vi "Get Waveform Queue Settings.vi"(1 "RT Data in":T1={"Device Ref"=18446744073709551615, "Waveforms"=[], "Channels"={"Command Chan Refs"=[], "Command Data Refs"=[], "Command Values"=[], "Status Chan Refs"=[], "Status Data Refs"=[], "Status Values"=[], "System Time"={"System Time"=timestamp(0 s since 1904-01-01), "Data Reference"=0, "Absolute Time Channel Data Ref"=0, "Get Date-Time Channel Data Ref"=0}, "Trigger Chan Refs"=[], "Trigger Data Refs"=[], "Trigger Values"=[]}, "Waveform Logs"=[], "Communication"={"Async Status"=refnum, "Wfm Comm Properties"={"WPL"={"Custom Queue Size"=1, "Use Custom Queue Size?"=FALSE}}, "Shutdown Event"=refnum, "Trigger Event"=refnum, "New File Event"=refnum, "Log Queues"=[], "Async VI Ref"=refnum}, "error"={"status"=FALSE, "code"=0, "source"=""}} {"Device Ref" format="%.0x"; "Channels"."Trigger Data Refs"."Data Reference" format="%.0x"; "Channels"."Trigger Chan Refs" format="%.0x"; "Channels"."System Time"."Get Date-Time Channel Data Ref" format="%.0x"; "Channels"."System Time"."Absolute Time Channel Data Ref" format="%.0x"; "Channels"."System Time"."Channel Data Reference" format="%.0x"; "Channels"."Status Data Refs"."Data Reference" format="%.0x"; "Channels"."Command Data Refs"."Data Reference" format="%.0x"; "Channels"."Status Chan Refs" format="%.0x"; "Channels"."Command Chan Refs" format="%.0x"; "Waveforms"."Waveform Ref in" format="%.0x"; "Waveform Logs"."Node ID" format="%.0x"; "Waveform Logs"."TDMS Error Code"."Data Ref" format="%.0x"; "Waveform Logs"."Missed Samples"."Data Ref" format="%.0x"; "Waveform Logs"."File Status"."Data Ref" format="%.0x"; "Waveform Logs"."Start New File"."Data Ref" format="%.0x"; "Waveform Logs"."Logging Enabled"."Data Ref" format="%.0x"; "Waveform Logs"."Stop Trigger"."Node Data Ref" format="%.0x"; "Waveform Logs"."Stop Trigger"."Node ID" format="%.0x"; "Waveform Logs"."Start Trigger"."Node Data Ref" format="%.0x"; "Waveform Logs"."Start Trigger"."Node ID" format="%.0x"}) -> (0 "RT Data out":T1={"Device Ref"=18446744073709551615, "Waveforms"=[], "Channels"={"Command Chan Refs"=[], "Command Data Refs"=[], "Command Values"=[], "Status Chan Refs"=[], "Status Data Refs"=[], "Status Values"=[], "System Time"={"System Time"=timestamp(0 s since 1904-01-01), "Data Reference"=0, "Absolute Time Channel Data Ref"=0, "Get Date-Time Channel Data Ref"=0}, "Trigger Chan Refs"=[], "Trigger Data Refs"=[], "Trigger Values"=[]}, "Waveform Logs"=[], "Communication"={"Async Status"=refnum, "Wfm Comm Properties"={"WPL"={"Custom Queue Size"=1, "Use Custom Queue Size?"=FALSE}}, "Shutdown Event"=refnum, "Trigger Event"=refnum, "New File Event"=refnum, "Log Queues"=[], "Async VI Ref"=refnum}, "error"={"status"=FALSE, "code"=0, "source"=""}} {"Device Ref" format="%.0x"; "Channels"."Trigger Data Refs"."Data Reference" format="%.0x"; "Channels"."Trigger Chan Refs" format="%.0x"; "Channels"."System Time"."Get Date-Time Channel Data Ref" format="%.0x"; "Channels"."System Time"."Absolute Time Channel Data Ref" format="%.0x"; "Channels"."System Time"."Channel Data Reference" format="%.0x"; "Channels"."Status Data Refs"."Data Reference" format="%.0x"; "Channels"."Command Data Refs"."Data Reference" format="%.0x"; "Channels"."Status Chan Refs" format="%.0x"; "Channels"."Command Chan Refs" format="%.0x"; "Waveforms"."Waveform Ref in" format="%.0x"; "Waveform Logs"."Node ID" format="%.0x"; "Waveform Logs"."TDMS Error Code"."Data Ref" format="%.0x"; "Waveform Logs"."Missed Samples"."Data Ref" format="%.0x"; "Waveform Logs"."File Status"."Data Ref" format="%.0x"; "Waveform Logs"."Start New File"."Data Ref" format="%.0x"; "Waveform Logs"."Logging Enabled"."Data Ref" format="%.0x"; "Waveform Logs"."Stop Trigger"."Node Data Ref" format="%.0x"; "Waveform Logs"."Stop Trigger"."Node ID" format="%.0x"; "Waveform Logs"."Start Trigger"."Node Data Ref" format="%.0x"; "Waveform Logs"."Start Trigger"."Node ID" format="%.0x"})   [LabVIEW 2015, in "Waveform Data Logger Engine.lvlib"]
uses:
  Waveform Data Logger Engine.lvlib
  Types/RT Data.ctl
  <vilib>/NI Veristand/Custom Device API/Custom Device Item Ref.ctl
  Types/Inline Waveform Info.ctl
  <vilib>/NI Veristand/Custom Device API/Waveform Data Reference.ctl
  Classes/Waveforms/Waveform Receive/Associated Log.ctl
  <vilib>/NI Veristand/Custom Device API/Custom Device Waveform DataType.ctl
  Types/Channels.ctl
  <vilib>/NI Veristand/Custom Device API/Block Data Reference.ctl
  <vilib>/NI Veristand/Custom Device API/Data Reference.ctl
  Types/System Time.ctl
  Types/Inline Waveform Log Info.ctl
  Shared/Classes/Log File Specifications/Waveform TDMS Log File Specification/Waveform TDMS Log File Specification.lvclass
  Classes/Triggers/Trigger/Trigger.lvclass
  Types/Inline Log Waveform.ctl
  Types/Trigger Settings.ctl
  Types/Log Status.ctl
  Types/Channel.ctl
  Types/Communication.ctl
  Types/Async Status.ctl
  Types/Async State.ctl
  <vilib>/NI Veristand/Custom Device Waveform API/Communication Properties.ctl
  Types/Trigger Event Data.ctl
  Types/Trigger Received.ctl
  Types/New File Event Data.ctl
  Types/Log Queues.ctl
  Shared/Globals/Property Strings.vi
  <vilib>/NI Veristand/Custom Device API/Get Item Property (I32).vi
  <vilib>/NI VeriStand/Custom Device API/Custom Device API.lvlib
  Shared/Waveform Data Logger Shared.lvlib
  Classes/Waveforms/Waveform Receive/Waveform Receive.lvclass
  <vilib>/NI Veristand/Custom Device Waveform API/NI_VS Custom Device Waveform API.lvlib
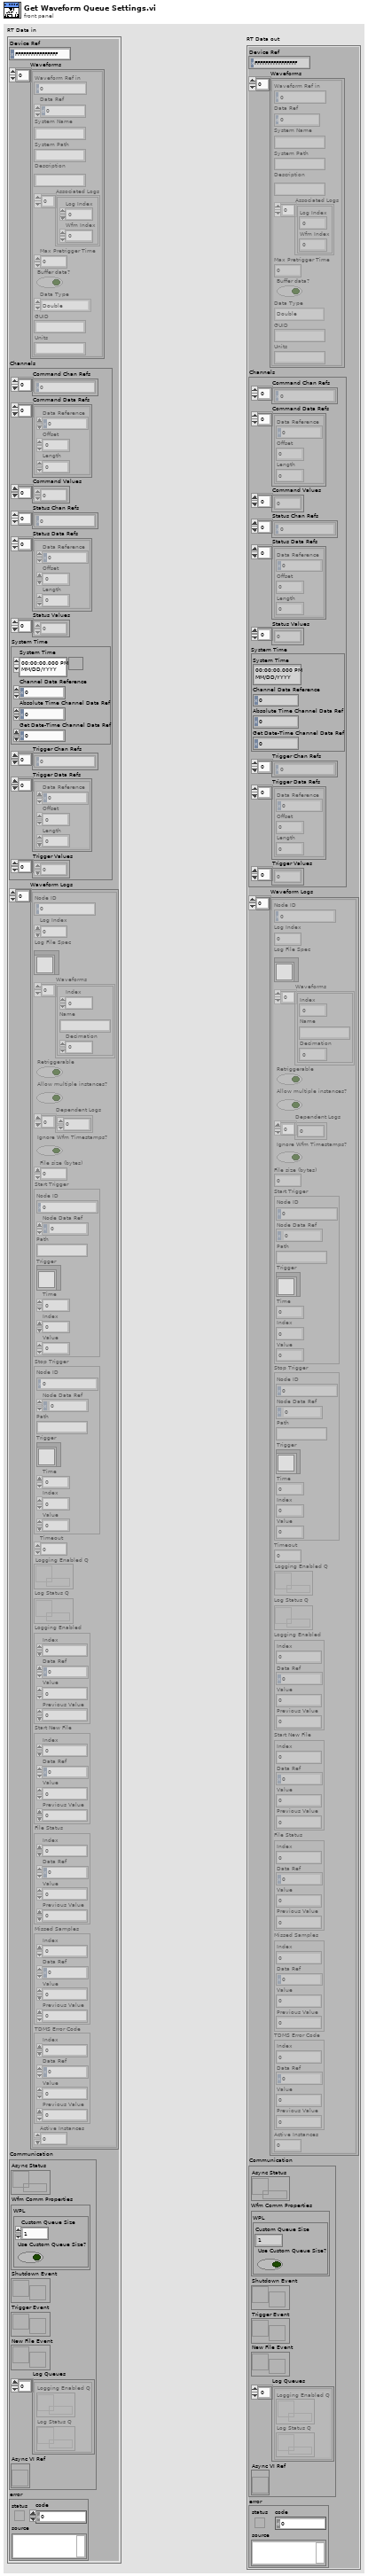
[diagram p1: front panel]
types:
  T1 = typedef "Waveform Data Logger Engine.lvlib/RT Data.ctl" = cluster{"Device Ref":T2, "Waveforms":T3[], "Channels":T7, "Waveform Logs":T11[], "Communication":T15, "error":errorcluster}
  T2 = typedef "Custom Device API.lvlib/Custom Device Item Ref.ctl" = u64
  T3 = typedef "Waveform Data Logger Engine.lvlib/Inline Waveform Info.ctl" = cluster{"Waveform Ref in":T2, "Data Ref":T4, "System Name":string, "System Path":string, "Description":string, "Associated Logs":T5[], "Max Pretrigger Time":dbl, "Buffer data?":bool, "Data Type":T6, "GUID":string, "Units":string}
  T4 = typedef "Custom Device API.lvlib/Waveform Data Reference.ctl" = i32
  T5 = typedef "Waveform Data Logger Engine.lvlib/Waveform Receive.lvclass/Associated Log.ctl" = cluster{"Log Index":i32, "Wfm Index":i32}
  T6 = typedef "Custom Device API.lvlib/Custom Device Waveform DataType.ctl" = enum16{"Double", "Complex Double"}
  T7 = typedef "Waveform Data Logger Engine.lvlib/Channels.ctl" = cluster{"Command Chan Refs":T2[], "Command Data Refs":T8[], "Command Values":dbl[], "Status Chan Refs":T2[], "Status Data Refs":T8[], "Status Values":dbl[], "System Time":T10, "Trigger Chan Refs":T2[], "Trigger Data Refs":T8[], "Trigger Values":dbl[]}
  T8 = typedef "Custom Device API.lvlib/Block Data Reference.ctl" = cluster{"Data Reference":T9, "Offset":u64, "Length":u64}
  T9 = typedef "Custom Device API.lvlib/Data Reference.ctl" = i32
  T10 = typedef "Waveform Data Logger Engine.lvlib/System Time.ctl" = cluster{"System Time":timestamp, "Data Reference":T9, "Absolute Time Channel Data Ref":T9, "Get Date-Time Channel Data Ref":T9}
  T11 = typedef "Waveform Data Logger Engine.lvlib/Inline Waveform Log Info.ctl" = cluster{"Node ID":T2, "Log Index":i32, "Log File Spec":refnum<class "Waveform TDMS Log File Specification.lvclass">, "Waveforms":T12[], "Retriggerable":bool, "Allow multiple instances?":bool, "Dependent Logs":i32[], "Ignore Wfm Timestamps?":bool, "File size (bytes)":i64, "Start Trigger":T13, "Stop Trigger":T13, "Timeout":dbl, "Logging Enabled Q":refnum<queue>, "Log Status Q":refnum<queue>, "Logging Enabled":T14, "Start New File":T14, "File Status":T14, "Missed Samples":T14, "TDMS Error Code":T14, "Active Instances":i32}
  T12 = typedef "Waveform Data Logger Engine.lvlib/Inline Log Waveform.ctl" = cluster{"Index":i32, "Name":string, "Decimation":u32}
  T13 = typedef "Waveform Data Logger Engine.lvlib/Trigger Settings.ctl" = cluster{"Node ID":T2, "Node Data Ref":i32, "Path":string, "Trigger":refnum<class "Trigger.lvclass">, "Time":dbl, "Index":i32, "Value":dbl}
  T14 = typedef "Waveform Data Logger Engine.lvlib/Channel.ctl" = cluster{"Index":i32, "Data Ref":T9, "Value":dbl, "Previous Value":dbl}
  T15 = typedef "Waveform Data Logger Engine.lvlib/Communication.ctl" = cluster{"Async Status":refnum<queue>, "Wfm Comm Properties":T16, "Shutdown Event":refnum<user-event>, "Trigger Event":refnum<user-event>, "New File Event":refnum<user-event>, "Log Queues":T17[], "Async VI Ref":refnum<vi>}
  T16 = typedef "NI_VS Custom Device Waveform API.lvlib/Communication Properties.ctl" = cluster{"WPL":cluster{"Custom Queue Size":i32, "Use Custom Queue Size?":bool}}
  T17 = typedef "Waveform Data Logger Engine.lvlib/Log Queues.ctl" = cluster{"Logging Enabled Q":refnum<queue>, "Log Status Q":refnum<queue>}
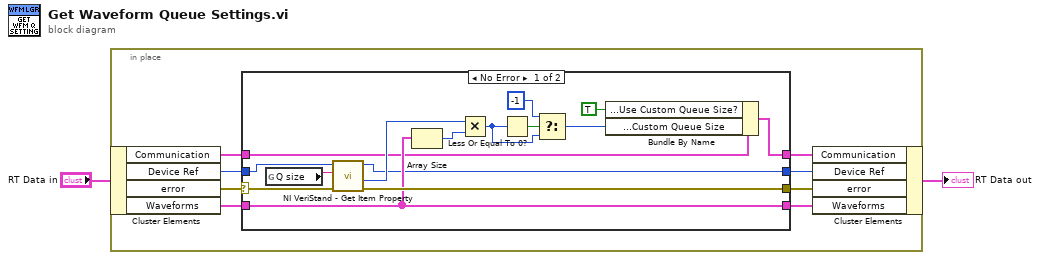
[diagram p0: block diagram]
diagram:
  n1 = in-place {
    n2 = in-place-cluster #1("RT Data in") -> ("Communication"=w7:T15, "Device Ref"=w8:T2, "error"=w10:errorcluster, "Waveforms"=w4:T3[])
    n3 = case shown="No Error" w10 {
      selector: w10 -> [w24 w29]
      tunnel: [w19 w29] -> w9
      tunnel: w8 -> [w23 w28]
      tunnel: w7 -> [w15 w27]
      tunnel: [w20 w27] -> w6
      tunnel: [w16 w28] -> w5
      tunnel: w4 -> [w18 w26]
      tunnel: [w18 w26] -> w3
      frame No Error {
        n4 = global read "Property Strings.vi" "Q size"() -> (w25:string)
        n5 = call-poly <vilib>:"NI VeriStand - Get Item Property.vi"("error in (no error)"=w24, "Property Name"=w25, "Item Ref in"=w23) -> ("error out"=w19:errorcluster, "Value"=w21:i32, "Item Ref out"=w16:T2)  [unwired: 5 in, 1 out]
        n6 = Array Size(array=w18) -> (size(s)=w22:i32)
        n7 = Multiply(x=w21, y=w22) -> (x*y=w13:i32)
        n8 = Less Or Equal To 0?(x=w13) -> (x <= 0?=w14:bool)
        n9 = Select(t=-1, s=w14, f=w13) -> (s? t:f=w12:i32)
        n10 = Bundle By Name(cluster=w15, "Wfm Comm Properties.WPL.Use Custom Queue Size?"=TRUE, "Wfm Comm Properties.WPL.Custom Queue Size"=w12) -> (w20:T15)
      }
      frame Error {
      }
    }
    n11 = in-place-cluster #1("Communication"=w6, "Device Ref"=w5, "error"=w9, "Waveforms"=w3) -> (→"RT Data out":T1)
  }
